vi "readArduino.vi"(8 "error in (no error)":errorcluster, 10 "String":string, 11 "reference":refnum<visa-resource-name>) -> (0 "error out":errorcluster, 2 "read buffer":string, 3 "VISA resource name out":refnum<visa-resource-name>)   [LabVIEW 2015]
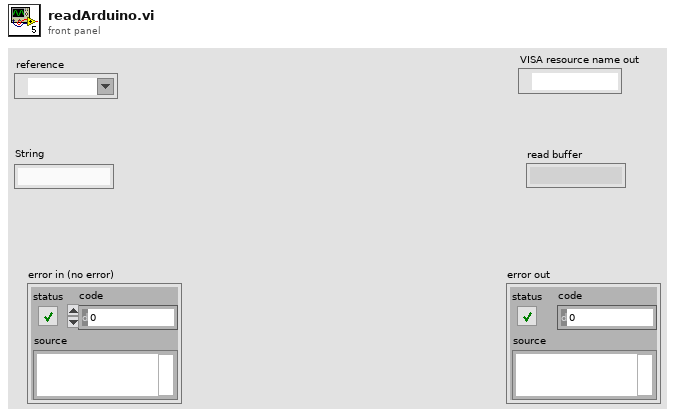
[diagram p1: front panel]
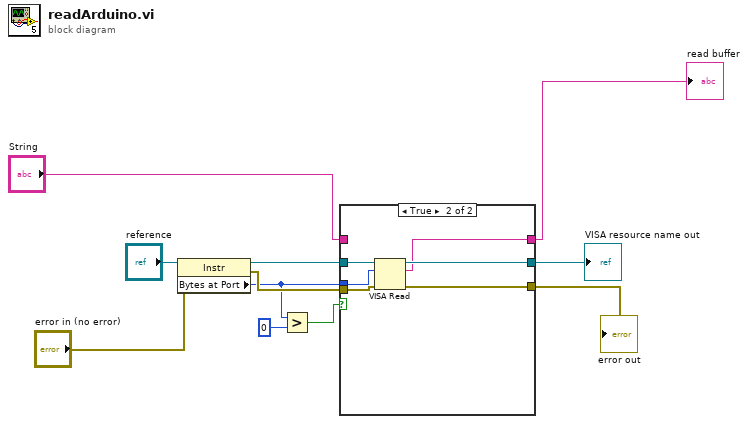
[diagram p0: block diagram]
diagram:
  n1 = property class="Instr"(reference="reference", error in="error in (no error)") -> (reference out=w9:refnum<visa-resource-name>, error out=w8:errorcluster, "Bytes at Port"=w5:u32)
  n2 = Greater?(x=w5, y=u32 0) -> (0:w6:bool)
  n3 = case shown="True" w6 {
    tunnel: w9 -> [w14 w20]
    tunnel: w5 -> [_ w19]
    tunnel: [w14 w18] -> w1
    tunnel: [w13 w17] -> w2
    tunnel: w8 -> [w13 w16]
    tunnel: [w12 w15] -> w7
    tunnel: "String" -> [w12 _]
    frame False {
    }
    frame True {
      n4 = VISA Read(VISA resource name=w20, byte count=w19, error in (no error)=w16) -> (VISA resource name out=w18:refnum<visa-resource-name>, read buffer=w15:string, error out=w17:errorcluster)  [unwired: 1 out]
    }
  }
  "read buffer" <- w7
  "VISA resource name out" <- w1
  "error out" <- w2
